vi "ABR3-Parse Data.vi"(0 "Data":dbl[](array[numeric]), 1 "Reject OverRide":bool, 2 "Rej Thresh µV":dbl=15.0, 7 "scale factor":dbl=1.0, 9 "Acquired In":i32, 11 "error in (no error)":errorcluster, 12 "Runtime":T1={"Ceiling"=0.0, "Threshold"=0.0, "Crossed?"=FALSE, "Step"=0, "Stop"=0, "Avgs"=0, "Level"=0.0, "AI Npts"=0, "Doubled?"=FALSE, "Gain"=0.0, "NWindowPts"=0, "dt"=0.0, "Cal"=path "", "Freq"=0.0, "AO Channels"=[], "AltPol"=FALSE, "AO Npts"=0, "AO Fs"=0.0, "Start"=0, "Stop max"=0, "Ear"=enum."Right", "Waveform"=enum."TONE PIP", "RepRate"=0.0, "CAP or ABR"=1, "LMasker"=0.0, "SeqVar"=enum."Signal Level", "Reps/buffer"=0, "Avg Mode"=enum."Neural/CM", "Wav"=path "", "Order"=enum."Sequential", "Levels"=[], "ControlVal"=0.0, "innerIndex"=0, "indexStep"=0} {"CAP or ABR" items=["CAP", "ABR"]}) -> (3 "Finished?":bool, 4 "Any rejected?":bool, 6 "RunSum1":dbl[](array[numeric]), 8 "RunSum2":dbl[](array[numeric]), 10 "Acquired Out":i32, 14 "Ntries":i32, 15 "error out":errorcluster)   [LabVIEW 2020]
uses:
  TypeDefs/ABR3-Runtime Data.ctl
  epl-vi-lib/Utility VIs/Type Defs/Left-Right ring.ctl
  TypeDefs/ABR-Waveform Enum.ctl
  TypeDefs/ABR3-Seq Var Enum.ctl
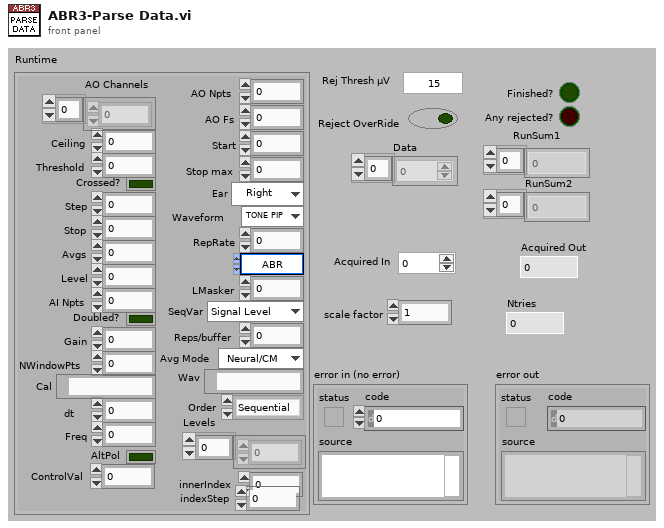
[diagram p1: front panel]
types:
  T1 = typedef "ABR3-Runtime Data.ctl" = cluster{"Ceiling":dbl, "Threshold":dbl, "Crossed?":bool, "Step":i32, "Stop":i32, "Avgs":i32, "Level":dbl, "AI Npts":i32, "Doubled?":bool, "Gain":dbl, "NWindowPts":i32, "dt":dbl, "Cal":path, "Freq":dbl, "AO Channels":i32[], "AltPol":bool, "AO Npts":i32, "AO Fs":dbl, "Start":i32, "Stop max":i32, "Ear":T2, "Waveform":T3, "RepRate":dbl, "CAP or ABR":u16, "LMasker":dbl, "SeqVar":T4, "Reps/buffer":i32, "Avg Mode":enum16{"Neural/CM", "ANOW"}, "Wav":path, "Order":enum16{"Sequential", "Random"}, "Levels":dbl[], "ControlVal":dbl, "innerIndex":i32, "indexStep":i32}
  T2 = typedef "Left-Right ring.ctl" = enum16{"Right", "Left"}
  T3 = typedef "ABR-Waveform Enum.ctl" = enum16{"TONE PIP", "CLICK", "FILE", "CHIRP", "NOISE", "VERHULST"}
  T4 = typedef "ABR3-Seq Var Enum.ctl" = enum16{"Signal Level", "Masker Level"}
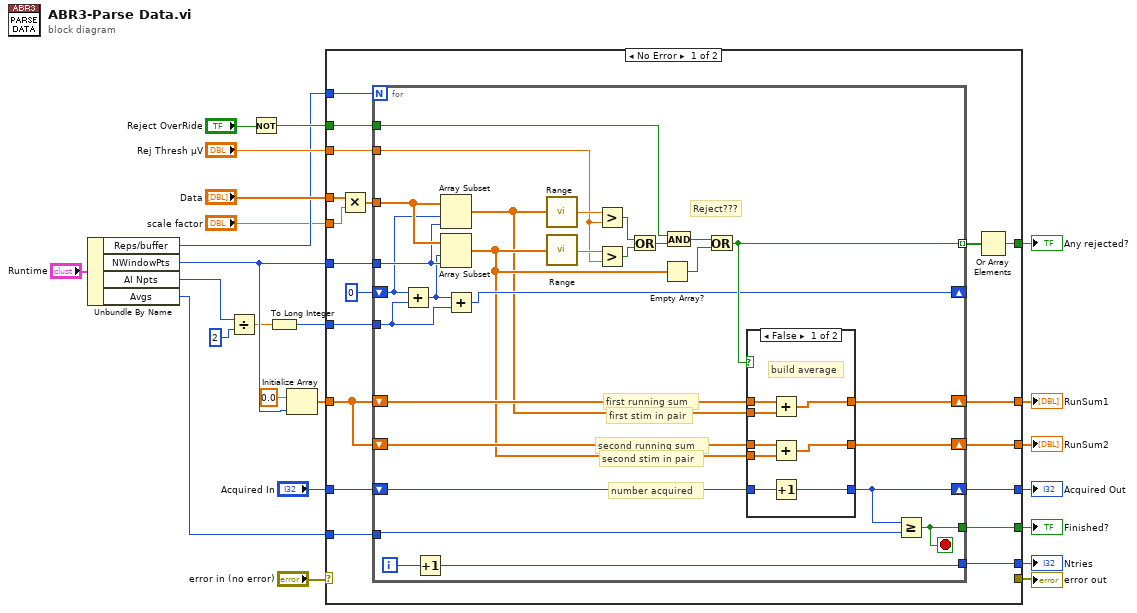
[diagram p0: block diagram]
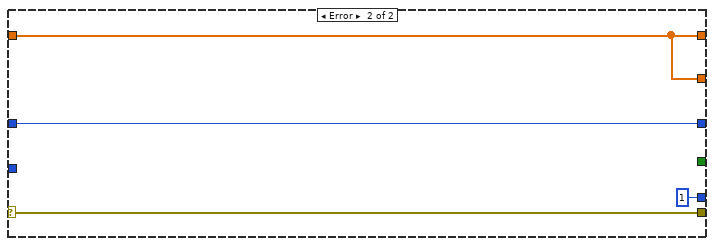
[diagram p3: hidden frame]
diagram:
  n1 = Unbundle By Name("Runtime") -> ("Reps/buffer"=w4:i32, "NWindowPts"=w12:i32, "AI Npts"=w11:i32, "Avgs"=w7:i32)
  n2 = Divide(x=w11, y=2) -> (x/y=w9:dbl)
  n3 = Not(x="Reject OverRide") -> (.not. x?=w20:bool)
  n4 = To Long Integer(number=w9) -> (32bit integer=w8:i32)
  n5 = Initialize Array(0.0 ("element"), w12) -> (w16:dbl[])
  n6 = case shown="No Error" "error in (no error)" {
    selector: "error in (no error)" -> [_ w86]
    tunnel: [_ w86] -> w23
    tunnel: "Data" -> [w43 _]
    tunnel: w20 -> [w42 _]
    tunnel: "Rej Thresh µV" -> [w41 _]
    tunnel: w12 -> [w40 _]
    tunnel: w4 -> [w39 _]
    tunnel: w8 -> [w38 _]
    tunnel: [w36 _] -> w17
    tunnel: w16 -> [w35 w84]
    tunnel: [w33 w84] -> w1
    tunnel: [w32 w84] -> w2
    tunnel: [w31 w85] -> w15
    tunnel: "Acquired In" -> [w30 w85]
    tunnel: w7 -> [w29 _]
    tunnel: [w28 _] -> w6
    tunnel: [w27 1] -> w5
    tunnel: "scale factor" -> [w25 _]
    frame No Error {
      n7 = Multiply(x=w43, y=w25) -> (x*y=w26:dbl[])
      n8 = for {
        N: w39 -> [_]
        tunnel: w26 -> [w64]
        tunnel: w42 -> [w63]
        tunnel: w41 -> [w62]
        tunnel: w40 -> [w61]
        tunnel: w38 -> [w52]
        tunnel: [w60] -> w37 mode=indexing
        shift-right: [w50] -> w31
        shift-left: w30 -> [w59]
        shift-right: [w57] -> w33
        shift-left: w35 -> [w58]
        shift-right: [w56] -> w32
        shift-left: w35 -> [w55]
        shift-right: [w51] -> _
        shift-left: 0 -> [w54]
        tunnel: w29 -> [w49]
        tunnel: [w48] -> w28
        tunnel: [w46] -> w27
        i -> [w47]
        stop <- w48 stop-if-true
        # "Reject???"
        # "second running sum"
        # "first running sum"
        # "second stim in pair"
        # "first stim in pair"
        # "number acquired"
        n9 = Add(x=w54, y=w52) -> (x+y=w53:i32)
        n10 = Increment(x=w47) -> (x+1=w46:i32)
        n11 = Array Subset(array=w64, index=w54, length=w61) -> (w44:dbl[])
        n12 = Array Subset(array=w64, index=w53, length=w61) -> (w45:dbl[])
        n13 = Add(x=w53, y=w52) -> (x+y=w51:i32)
        n14 = call "Range.vi"("Array"=w44) -> ("Range"=w66:dbl)
        n15 = call "Range.vi"("Array"=w45) -> ("Range"=w65:dbl)
        n16 = Greater?(x=w66, y=w62) -> (0:w68:bool)
        n17 = Greater?(x=w65, y=w62) -> (0:w67:bool)
        n18 = Or(x=w68, y=w67) -> (x .or. y?=w69:bool)
        n19 = Empty Array?(array=w45) -> (empty?=w70:bool)
        n20 = And(x=w63, y=w69) -> (x .and. y?=w71:bool)
        n21 = Or(x=w71, y=w70) -> (x .or. y?=w60:bool)
        n22 = case shown="False" w60 {
          tunnel: w44 -> [w77 _]
          tunnel: w45 -> [w73 _]
          tunnel: w59 -> [w79 w82]
          tunnel: [w78 w82] -> w50
          tunnel: w58 -> [w76 w81]
          tunnel: [w75 w81] -> w57
          tunnel: [w74 w80] -> w56
          tunnel: w55 -> [w72 w80]
          frame False {
            # "build average"
            n23 = Add(x=w76, y=w77) -> (x+y=w75:dbl[])
            n24 = Add(x=w72, y=w73) -> (x+y=w74:dbl[])
            n25 = Increment(x=w79) -> (x+1=w78:i32)
          }
          frame True {
          }
        }
        n26 = Greater Or Equal?(x=w50, y=w49) -> (x >= y?=w48:bool)
      }
      n27 = Or Array Elements(Boolean array=w37) -> (logical OR=w36:bool)
    }
    frame Error {
    }
  }
  "error out" <- w23
  "Any rejected?" <- w17
  "RunSum1" <- w1
  "RunSum2" <- w2
  "Acquired Out" <- w15
  "Finished?" <- w6
  "Ntries" <- w5
